vi "examenParcial1_520.vi"() -> ()   [LabVIEW 2011]
panel:
  out "temp>32":dbl
  out "TempPromedio":dbl
  out "TempMenor":dbl
  out "TempMayor":dbl
  out "temp>32":bool
  out "30-50":bool
  out "21-30":bool
  out "1-20":bool
  out "Temperatura":i32(slide) scale=0.0..50.0
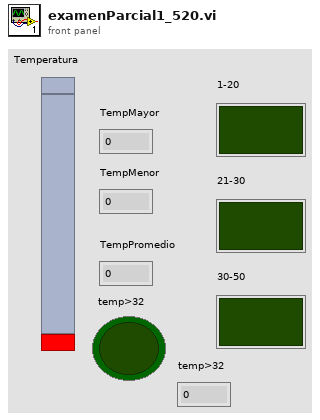
[diagram p1: front panel]
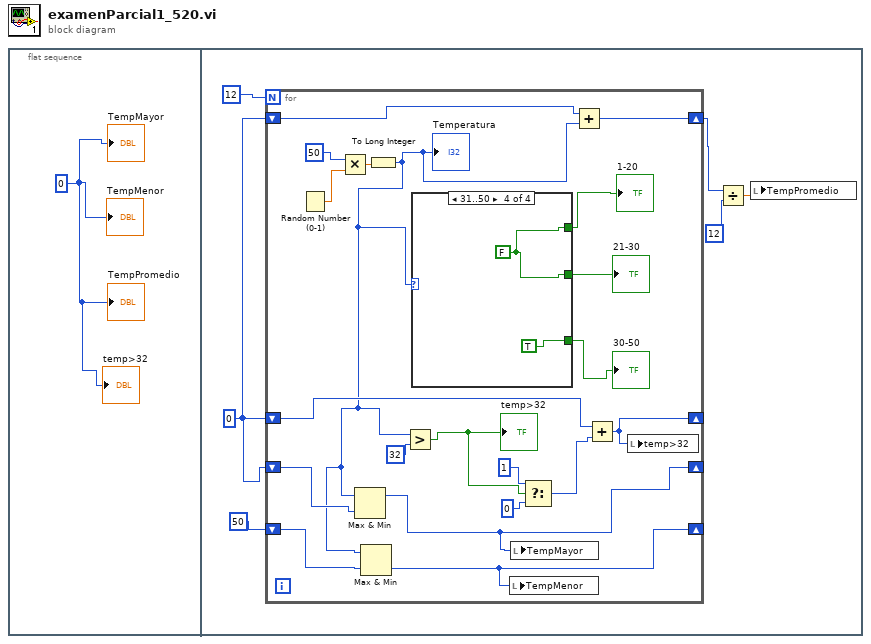
[diagram p0: block diagram]
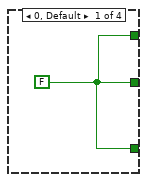
[diagram p2: hidden frame]
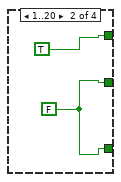
[diagram p3: hidden frame]
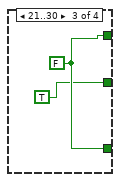
[diagram p4: hidden frame]
diagram:
  n1 = flat-sequence {
    frame #0 {
      w1 = 0
      "TempMayor" <- w1
      "TempMenor" <- w1
      "TempPromedio" <- w1
      "temp>32" <- w1
    }
    frame #1 {
      w5 = 0
      n2 = for {
        N: 12 -> [_]
        shift-right: [w15] -> _
        shift-left: w5 -> [w20]
        shift-right: [w11] -> _
        shift-left: w5 -> [w14]
        shift-right: [w12] -> _
        shift-left: 50 -> [w13]
        shift-right: [w8] -> w4
        shift-left: w5 -> [w10]
        n3 = Random Number (0-1)() -> (number: 0 to 1=w26:dbl)
        n4 = Multiply(x=50, y=w26) -> (x*y=w25:dbl)
        n5 = To Long Integer(number=w25) -> (32bit integer=w9:i32)
        "Temperatura" <- w9
        n6 = Max & Min(x=w9, y=w14) -> (max(x,y)=w11:i32)  [unwired: 1 out]
        n7 = Max & Min(x=w9, y=w13) -> (min(x,y)=w12:i32)  [unwired: 1 out]
        n8 = Greater?(x=w9, y=32) -> (0:w19:bool)
        "temp>32" <- w19
        n9 = case shown="31..50" w9 {
          tunnel: [w28 TRUE w32 w33] -> w24
          tunnel: [w28 w29 w32 TRUE] -> w23
          tunnel: [w28 w29 TRUE w33] -> w22
          frame 0, Default {
            w28 = FALSE
          }
          frame 1..20 {
            w29 = FALSE
          }
          frame 21..30 {
            w32 = FALSE
          }
          frame 31..50 {
            w33 = FALSE
          }
        }
        "1-20" <- w24
        "21-30" <- w22
        "30-50" <- w23
        n10 = local write "TempMenor"(w12) -> ()
        n11 = local write "TempMayor"(w11) -> ()
        n12 = Select(t=1, s=w19, f=0) -> (s? t:f=w16:i32)
        n13 = Add(x=w10, y=w9) -> (x+y=w8:i32)
        n14 = Add(x=w20, y=w16) -> (x+y=w15:i32)
        n15 = local write "temp>32"(w15) -> ()
      }
      n16 = Divide(x=w4, y=12) -> (x/y=w2:dbl)
      n17 = local write "TempPromedio"(w2) -> ()
    }
  }
